vi "Decorator.vi"(8 "error in (no error)":errorcluster, 10 "DecoratorData in":refnum<class "Data.lvclass">, 11 "DataVer2 in":refnum<class "DataVer2.lvclass">) -> (0 "error out":errorcluster, 3 "DataVer2 out":refnum<class "DataVer2.lvclass">)   [LabVIEW 2013, in "DataVer2.lvclass"]
uses:
  DataVer2.lvclass
  Data.lvclass/Data.lvclass
  DataVer2.lvclass/DataVer2.ctl
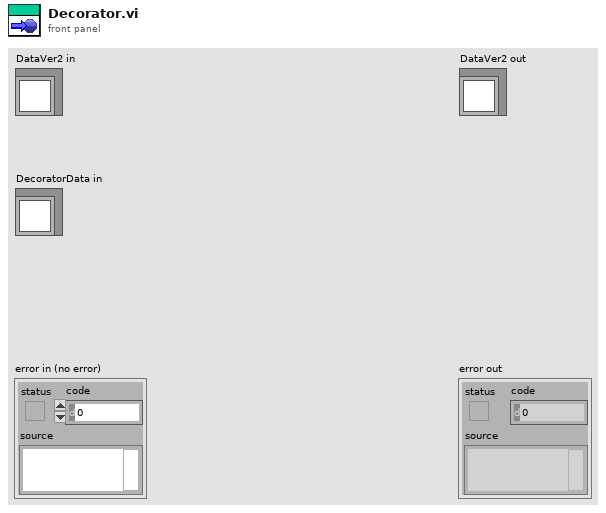
[diagram p1: front panel]
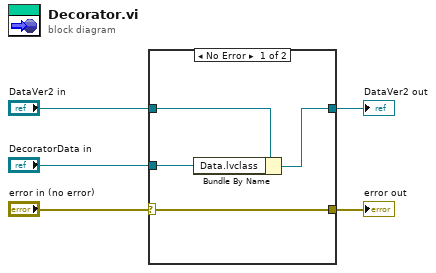
[diagram p0: block diagram]
diagram:
  n1 = case shown="No Error" "error in (no error)" {
    selector: "error in (no error)" -> [w9 w11]
    tunnel: [w9 w11] -> w3
    tunnel: [w6 w10] -> w4
    tunnel: "DataVer2 in" -> [w7 w10]
    tunnel: "DecoratorData in" -> [w8 _]
    frame No Error {
      n2 = Bundle By Name(cluster=w7, "Data.lvclass"=w8) -> (w6:refnum<class "DataVer2.lvclass">)
    }
    frame Error {
    }
  }
  "error out" <- w3
  "DataVer2 out" <- w4
